vi "licz_zakres.vi"(9 "x3":cdb, 10 "x2":cdb, 11 "x1":cdb) -> (2 "lewy zakres":dbl, 3 "prawy zakres":dbl)   [LabVIEW 2020]
doc: "Liczenie zakresu do wykresu +/-30%"
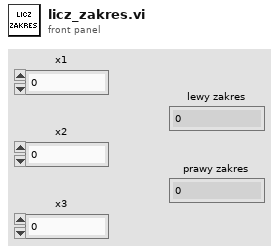
[diagram p1: front panel]
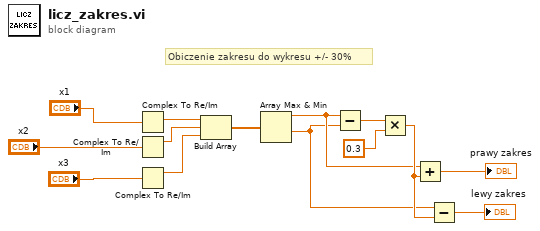
[diagram p0: block diagram]
diagram:
  # "Obiczenie zakresu do wykresu +/- 30%"
  n1 = Complex To Re/Im(x + iy="x1") -> (x=w4:dbl)  [unwired: 1 out]
  n2 = Complex To Re/Im(x + iy="x2") -> (x=w5:dbl)  [unwired: 1 out]
  n3 = Complex To Re/Im(x + iy="x3") -> (x=w6:dbl)  [unwired: 1 out]
  n4 = Build Array(w4, w5, w6) -> (w7:dbl[])
  n5 = Array Max & Min(array=w7) -> (max value=w11:dbl, min value=w10:dbl)  [unwired: 2 out]
  n6 = Subtract(x=w11, y=w10) -> (x-y=w8:dbl)
  n7 = Multiply(x=w8, y=0.3) -> (x*y=w12:dbl)
  n8 = Add(x=w11, y=w12) -> (x+y=→"prawy zakres":dbl)
  n9 = Subtract(x=w10, y=w12) -> (x-y=→"lewy zakres":dbl)
